vi "General Setup.vi"(9 "measurement mode":T1 {"gain" max=15}, 10 "setup":T2={"integration time"=0.5, "rinse time"=10.0, "sample time"=10.0, "sample type"=0} {"sample type" items=["Sample Cuvet", "Sipper Cell", "No Dialog"]; "sample time" min=0.0 max=100.0 step=1.0 format="%.1f"; "rinse time" min=0.0 max=100.0 step=1.0 format="%.1f"; "integration time" format="%.1f"}, 11 "GPIB in":string="18") -> (3 "GPIB out":string="18")   [LabVIEW 2015]
uses:
  settings.ctl
  measurement mode.ctl
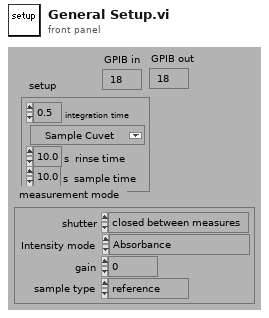
[diagram p1: front panel]
types:
  T1 = typedef "measurement mode.ctl" = cluster{"shutter":enum16{"closed between measures", "open between measures"}, "Intensity mode":enum16{"Absorbance", "Intensity at current gain", "Intensity at fixed gain", "dark current at current gain", "dark current at fixed gain"}, "gain":u8, "sample type":enum16{"reference", "standard", "unknown", "Diagnostic"}}
  T2 = typedef "settings.ctl" = cluster{"integration time":sgl, "rinse time":dbl[unit], "sample time":dbl[unit], "sample type":u16}
  T3 = enum16{"closed between measures", "open between measures"}
  T4 = enum16{"Absorbance", "Intensity at current gain", "Intensity at fixed gain", "dark current at current gain", "dark current at fixed gain"}
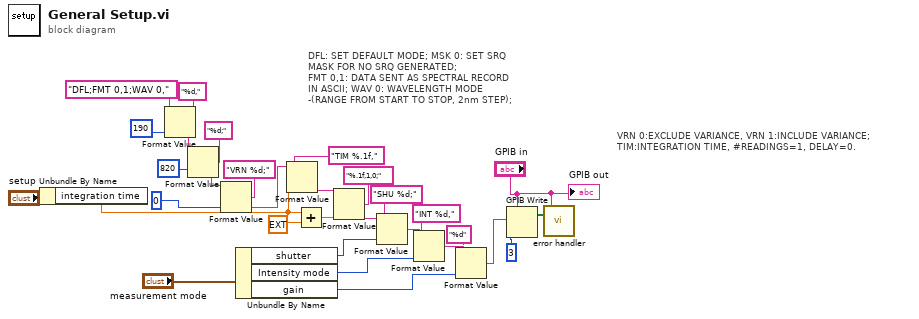
[diagram p0: block diagram]
diagram:
  # "VRN 0:EXCLUDE VARIANCE, VRN 1:INCLUDE VARIANCE;\nTIM:INTEGRATION TIME, #READINGS=1, DELAY=0."
  # "DFL: SET DEFAULT MODE; MSK 0: SET SRQ\nMASK FOR NO SRQ GENERATED;\nFMT 0,1: DATA SENT AS SPECTRAL RECORD\nIN ASCII; WAV 0: WAVELENGTH MODE\n-(RANGE FROM START TO STOP, 2nm STEP);"
  n1 = Unbundle By Name("setup") -> ("integration time"=w17:sgl)
  n2 = Format Value(string ("")="DFL;FMT 0,1;WAV 0,", format string="%d,", value (0)=190) -> (output string=w29:string)
  n3 = Format Value(string ("")=w29, format string="%d;", value (0)=820) -> (output string=w27:string)
  n4 = Format Value(string ("")=w27, format string="VRN %d;", value (0)=0) -> (output string=w24:string)
  n5 = Unbundle By Name("measurement mode") -> ("shutter"=w6:T3, "Intensity mode"=w5:T4, "gain"=w4:u8)
  n6 = Format Value(string ("")=w24, format string="TIM %.1f,", value (0)=w17) -> (output string=w22:string)
  n7 = Add(x=w17, y=ext 0.5) -> (x+y=w20:ext)
  n8 = Format Value(string ("")=w22, format string="%.1f,1,0;", value (0)=w20) -> (output string=w15:string)
  n9 = Format Value(string ("")=w15, format string="SHU %d;", value (0)=w6) -> (output string=w13:string)
  n10 = Format Value(string ("")=w13, format string="INT %d,", value (0)=w5) -> (output string=w12:string)
  n11 = Format Value(string ("")=w12, format string="%d", value (0)=w4) -> (output string=w10:string)
  n12 = GPIB Write(0:"GPIB in", 1:w10, 2:3) -> (5:w18:bool[])  [unwired: 2 in, 1 out]
  n13 = call "error handler.vi"("status array"=w18, "GPIB in"="GPIB in") -> ()  [unwired: 3 in, 3 out]
  "GPIB out" <- "GPIB in"
